vi "Check Closed Loop.vi"(9 "Answer":i32) -> (2 "Bit 0":bool, 3 "Output string":string)   [LabVIEW 2021]
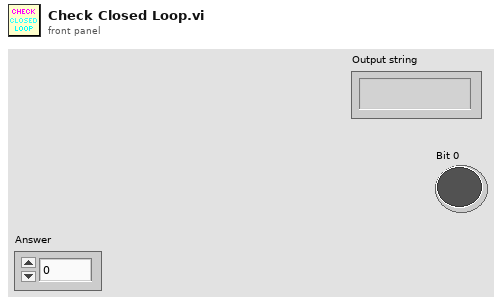
[diagram p1: front panel]
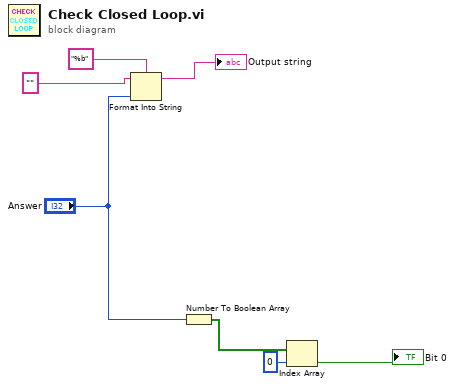
[diagram p0: block diagram]
diagram:
  n1 = Format Into String(format string="%b" ("initial string"), initial string="", "Answer") -> (resulting string=→"Output string":string)  [unwired: 1 in, 1 out]
  n2 = Number To Boolean Array(number="Answer") -> (Boolean array=w4:bool[])
  n3 = Index Array(array=w4, index=0) -> (element=→"Bit 0":bool)
